vi "Filter Values.vi"(8 "max rate":dbl, 10 "y-axis in":dbl, 11 "x-axis in":dbl) -> (2 "y-axis out":dbl, 3 "x-axis out":dbl)   [LabVIEW 2012]
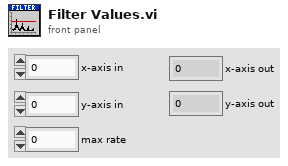
[diagram p1: front panel]
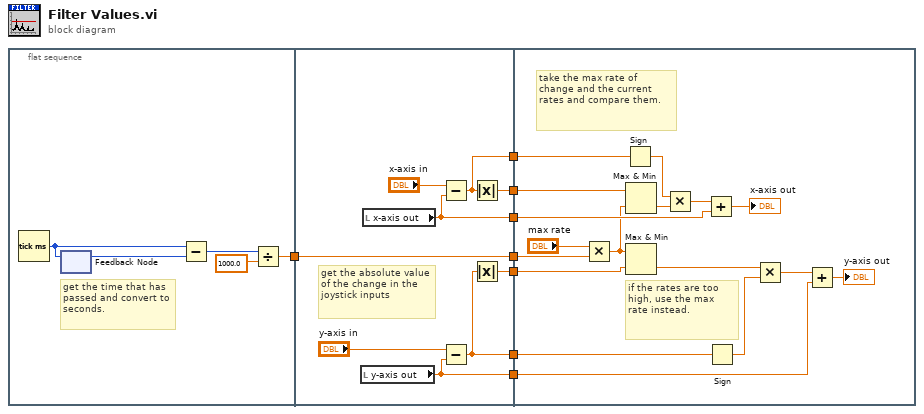
[diagram p0: block diagram]
diagram:
  n1 = flat-sequence {
    tunnel: [w9] -> w8
    tunnel: w8 -> [w14]
    tunnel: [w20] -> w7
    tunnel: [w19] -> w6
    tunnel: [w18] -> w5
    tunnel: [w17] -> w4
    tunnel: [w16] -> w3
    tunnel: [w15] -> w2
    tunnel: [w14] -> w1
    tunnel: w7 -> [w26]
    tunnel: w6 -> [w33]
    tunnel: w5 -> [w32]
    tunnel: w4 -> [w31]
    tunnel: w3 -> [w29]
    tunnel: w2 -> [w28]
    tunnel: w1 -> [w24]
    frame #0 {
      # "get the time that has passed and convert to seconds."
      n2 = Tick Count (ms)() -> (millisecond timer value=w12:u32)
      n3 = feedback #1() -> (w13:u32)  [unwired: 1 in]
      n4 = feedback-in #1(w12) -> ()
      n5 = Subtract(x=w12, y=w13) -> (x-y=w10:u32)
      n6 = Divide(x=w10, y=1000.0) -> (x/y=w9:dbl)
    }
    frame #1 {
      # "get the absolute value of the change in the joystick inputs"
      n7 = local read "y-axis out"() -> (w16:dbl)
      n8 = local read "x-axis out"() -> (w15:dbl)
      n9 = Subtract(x="x-axis in", y=w15) -> (x-y=w18:dbl)
      n10 = Subtract(x="y-axis in", y=w16) -> (x-y=w17:dbl)
      n11 = Absolute Value(x=w18) -> (abs(x)=w20:dbl)
      n12 = Absolute Value(x=w17) -> (abs(x)=w19:dbl)
    }
    frame #2 {
      # "if the rates are too high, use the max rate instead."
      # "take the max rate of change and the current rates and compare them."
      n13 = Multiply(x="max rate", y=w24) -> (x*y=w23:dbl)
      n14 = Sign(1:w32) -> (0:w36:dbl)
      n15 = Max & Min(x=w26, y=w23) -> (min(x,y)=w38:dbl)  [unwired: 1 out]
      n16 = Max & Min(x=w23, y=w33) -> (min(x,y)=w34:dbl)  [unwired: 1 out]
      n17 = Multiply(x=w36, y=w38) -> (x*y=w39:dbl)
      n18 = Add(x=w39, y=w28) -> (x+y=→"x-axis out":dbl)
      n19 = Sign(1:w31) -> (0:w35:dbl)
      n20 = Multiply(x=w34, y=w35) -> (x*y=w30:dbl)
      n21 = Add(x=w30, y=w29) -> (x+y=→"y-axis out":dbl)
    }
  }
